vi "comm write mode.vi"(5 "End of Transmission":string, 7 "Start of Transmission":string, 8 "error in (no error)":errorcluster, 9 "End of Transmission Enable":bool, 10 "Start of Transmission Enable":bool, 11 "Comm Handle":u32) -> (0 "error out":errorcluster, 3 "dup Comm Handle":u32)   [LabVIEW 2013, in "lvserial.lvlib"]
doc: "Configures the write mode. The transmission of a start of transmission and/or end of transmission string."
uses:
  lvserial.lvlib
  lvserial.dll
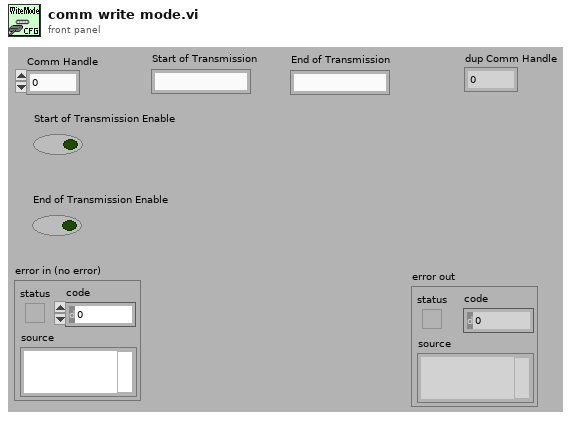
[diagram p1: front panel]
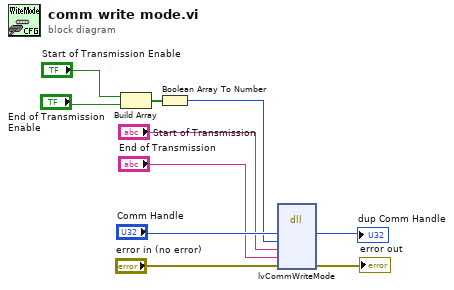
[diagram p0: block diagram]
diagram:
  n1 = Build Array("Start of Transmission Enable", "End of Transmission Enable") -> (w5:bool[])
  n2 = Boolean Array To Number(Boolean array=w5) -> (number=w1:u32)
  n3 = dll-call lib="lvserial.dll" fn="lvCommWriteMode"("hComm"="Comm Handle", "lWriteMode"=w1, "shStartOfTransmission"="Start of Transmission", "shEndOfTransmission"="End of Transmission", "error in (no error)"="error in (no error)") -> ("hComm"=→"dup Comm Handle":u32, "error in (no error)"=→"error out":errorcluster)  [unwired: 6 in, 3 out]
